vi "General Delay Codification.vi"(8 "Delay":dbl max=32767.0 step=1.0, 9 "ms/us Delay":bool) -> (0 "Final array":bool[](array[boolean]), 1 "Real Time":ext)   [LabVIEW 2011]
panel:
  out "hex integer string":string
  out "Time Error":ext
  out "Aprox Loops":ext
  out "Pure Loops":ext
  in  "fixed-point type":fxp<+,15,15>
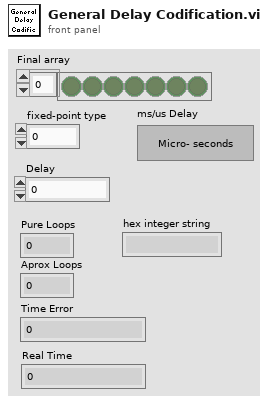
[diagram p1: front panel]
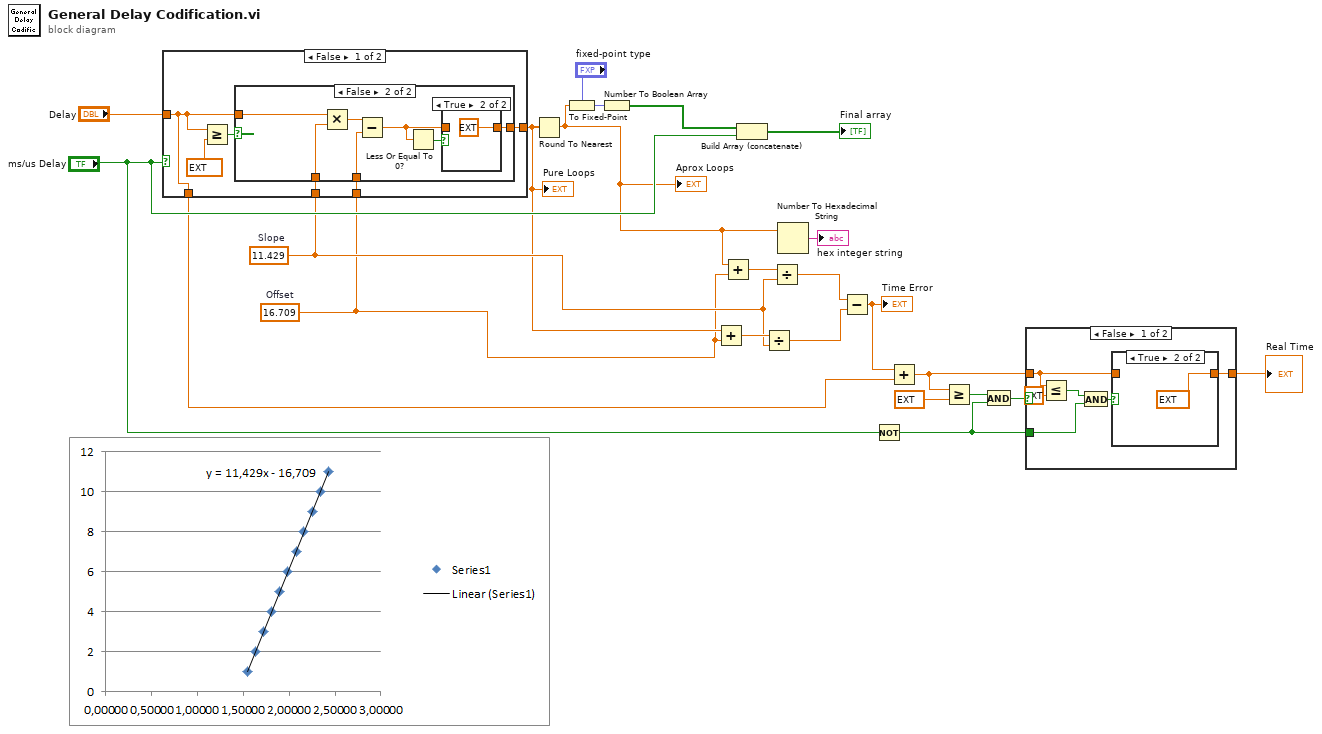
[diagram p0: block diagram]
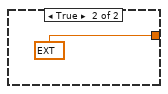
[diagram p3: hidden frame]
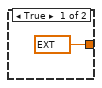
[diagram p4: hidden frame]
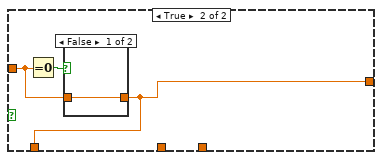
[diagram p6: hidden frame]
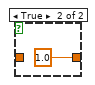
[diagram p7: hidden frame]
diagram:
  w2 = 16.709  # Offset
  w4 = 11.429  # Slope
  n1 = case shown="False" "ms/us Delay" {
    tunnel: "Delay" -> [w24 w41]
    tunnel: [w27 w40] -> w3
    tunnel: w4 -> [w26 _]
    tunnel: w2 -> [w25 _]
    tunnel: [w24 w40] -> w1
    frame False {
      n2 = Greater Or Equal?(x=w24, y=ext 1000.0) -> (x >= y?=w28:bool)
      n3 = case shown="False" w28 {
        tunnel: w24 -> [_ w37]
        tunnel: [ext 11422.0 w34] -> w27
        tunnel: w26 -> [_ w32]
        tunnel: w25 -> [_ w31]
        frame True {
        }
        frame False {
          n4 = Multiply(x=w37, y=w32) -> (x*y=w36:dbl)
          n5 = Subtract(x=w36, y=w31) -> (x-y=w33:dbl)
          n6 = Less Or Equal To 0?(x=w33) -> (x <= 0?=w35:bool)
          n7 = case shown="True" w35 {
            tunnel: [w38 ext 0.0] -> w34
            tunnel: w33 -> [w38 _]
            frame False {
            }
            frame True {
            }
          }
        }
      }
    }
    frame True {
      n8 = Equal To 0?(x=w41) -> (x = 0?=w42:bool)
      n9 = case shown="False" w42 {
        tunnel: [w43 1.0] -> w40
        tunnel: w41 -> [w43 _]
        frame False {
        }
        frame True {
        }
      }
    }
  }
  "Pure Loops" <- w3
  n10 = Round To Nearest(number=w3) -> (nearest integer value=w6:ext)
  "Aprox Loops" <- w6
  n11 = To Fixed-Point(fixed-point type="fixed-point type", number=w6) -> (fixed-point=w22:fxp<+,15,15>)
  n12 = Number To Boolean Array(number=w22) -> (Boolean array=w21:bool[])
  n13 = Add(x=w3, y=w2) -> (x+y=w18:ext)
  n14 = Add(x=w6, y=w2) -> (x+y=w19:ext)
  n15 = Build Array (concatenate)(w21, "ms/us Delay") -> (→"Final array":bool[])
  n16 = Divide(x=w18, y=w4) -> (x/y=w16:ext)
  n17 = Divide(x=w19, y=w4) -> (x/y=w17:ext)
  n18 = Number To Hexadecimal String(2:w6) -> (0:→"hex integer string":string)  [unwired: 1 in]
  n19 = Subtract(x=w17, y=w16) -> (x-y=w14:ext)
  "Time Error" <- w14
  n20 = Not(x="ms/us Delay") -> (.not. x?=w7:bool)
  n21 = Add(x=w14, y=w1) -> (x+y=w13:ext)
  n22 = Greater Or Equal?(x=w13, y=ext 1000.0) -> (x >= y?=w10:bool)
  n23 = And(x=w10, y=w7) -> (x .and. y?=w11:bool)
  n24 = case shown="False" w11 {
    tunnel: w13 -> [w47 _]
    tunnel: [w48 ext 1000.0] -> w8
    tunnel: w7 -> [w50 _]
    frame False {
      n25 = Less Or Equal?(x=w47, y=ext 1.0) -> (x <= y?=w45:bool)
      n26 = And(x=w45, y=w50) -> (x .and. y?=w49:bool)
      n27 = case shown="True" w49 {
        tunnel: w47 -> [w51 _]
        tunnel: [w51 ext 1.462] -> w48
        frame False {
        }
        frame True {
        }
      }
    }
    frame True {
    }
  }
  "Real Time" <- w8
